vi "TextDiff.vi"(8 "error in (no error)":errorcluster, 9 "Output Folders":T5, 10 "VI 2 Screenshots in":T1, 11 "VI 1 Screenshots in":T1) -> (0 "error out":errorcluster, 2 "Description":string, 3 "appended path":path)   [LabVIEW 2020, in "VIDiffScreenshots.lvlib"]
uses:
  VIDiffScreenshots.lvlib
  Utilities/Output Folders.ctl
  VIScreenshots.ctl
  ScreenshotInfo.ctl
  Screenshot Type.ctl
  Utilities/FilePaths.ctl
  Utilities/VIDiffUtilities.lvlib
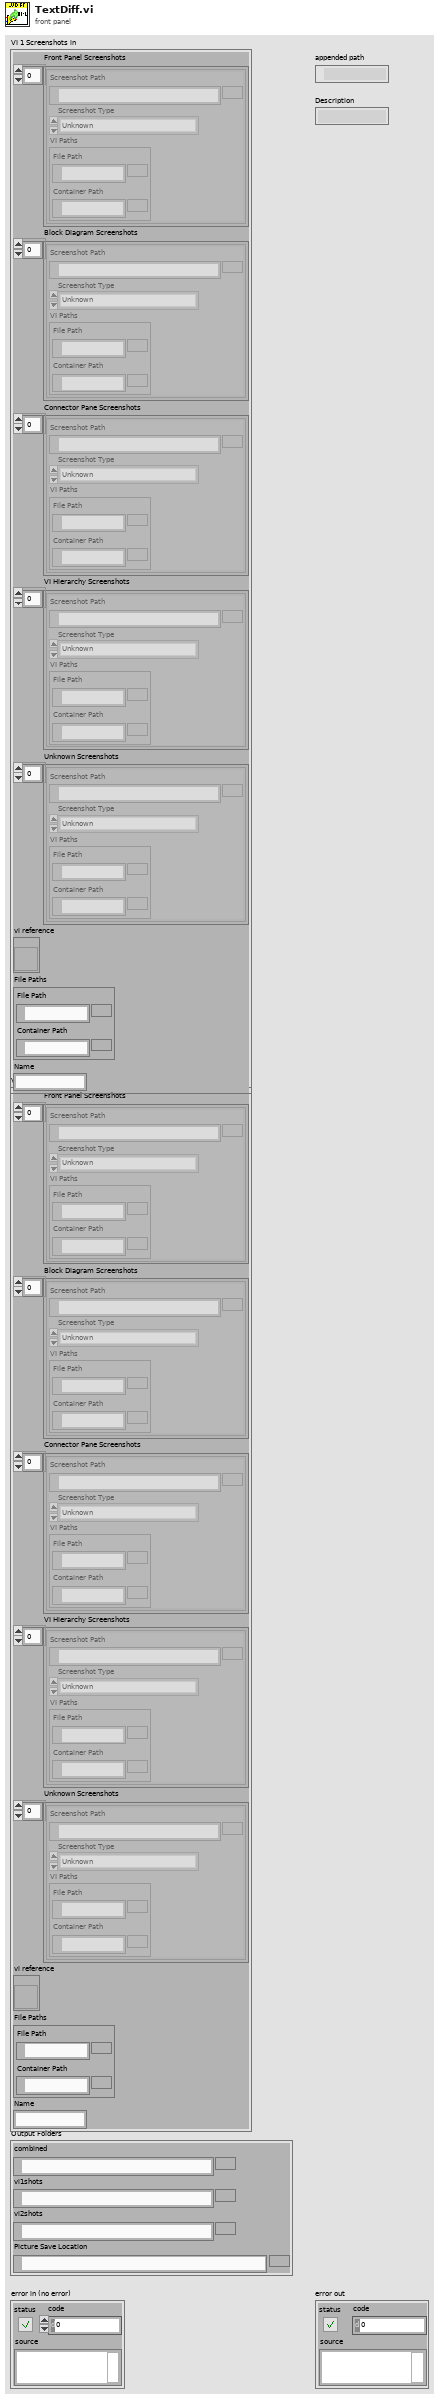
[diagram p1: front panel]
types:
  T1 = typedef "VIDiffScreenshots.lvlib/VIScreenshots.ctl" = cluster{"Front Panel Screenshots":T2[], "Block Diagram Screenshots":T2[], "Connector Pane Screenshots":T2[], "VI Hierarchy Screenshots":T2[], "Unknown Screenshots":T2[], "vi reference":refnum<vi>, "File Paths":cluster{"File Path":path, "Container Path":path}, "Name":string}
  T2 = typedef "VIDiffScreenshots.lvlib/ScreenshotInfo.ctl" = cluster{"Screenshot Path":path, "Screenshot Type":T3, "VI Paths":T4}
  T3 = typedef "VIDiffScreenshots.lvlib/Screenshot Type.ctl" = enum16{"Unknown", "Front Panel", "Connector Pane", "Block Diagram", "VI Hierarchy"}
  T4 = typedef "VIDiffUtilities.lvlib/FilePaths.ctl" = cluster{"File Path":path, "Container Path":path}
  T5 = typedef "VIDiffUtilities.lvlib/Output Folders.ctl" = cluster{"combined":path, "vi1shots":path, "vi2shots":path, "Picture Save Location":path}
  T6 = enum32{"invalid lock state", "Not Locked", "Locked (No Password)", "Password-protected"}
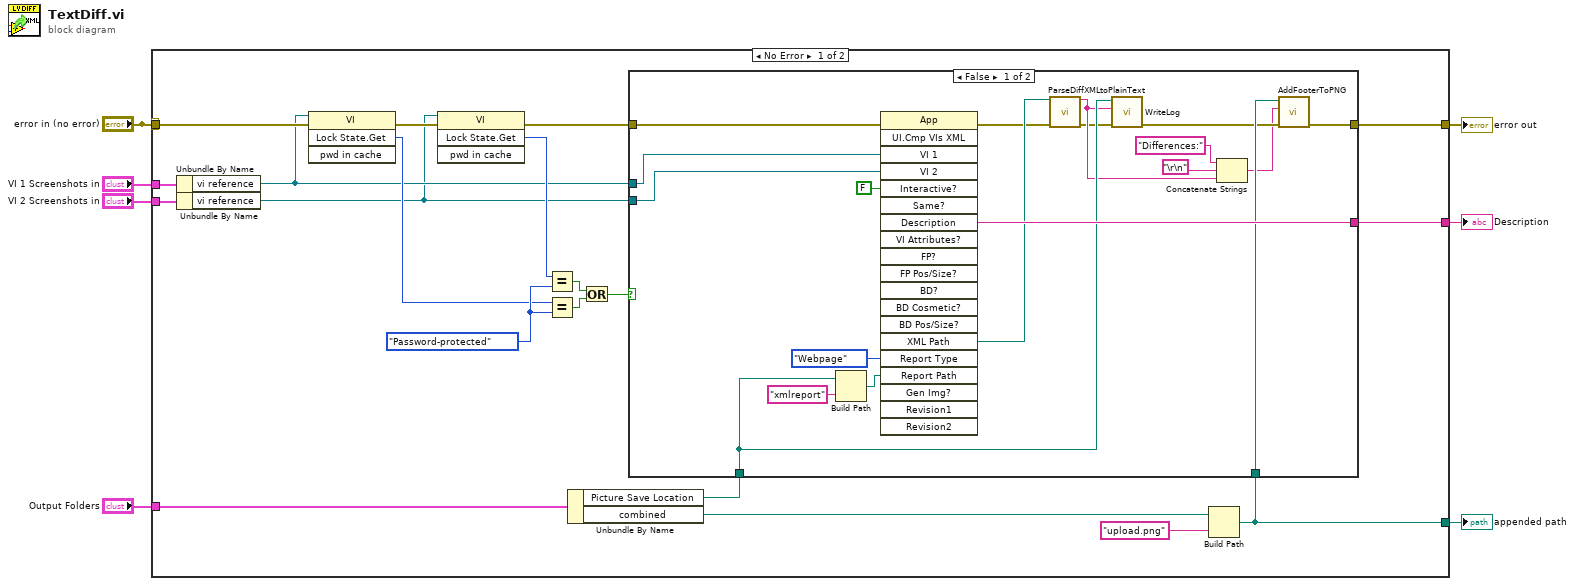
[diagram p0: block diagram]
diagram:
  n1 = case shown="No Error" "error in (no error)" {
    selector: "error in (no error)" -> [w21 w48]
    tunnel: "Output Folders" -> [w27 _]
    tunnel: "VI 2 Screenshots in" -> [w26 _]
    tunnel: "VI 1 Screenshots in" -> [w25 _]
    tunnel: "error in (no error)" -> [_ _]
    tunnel: [w24 _] -> w4
    tunnel: [w23 _] -> w3
    tunnel: [w22 w48] -> w2
    frame No Error {
      w18 = T6."Password-protected" ("y")
      n2 = Unbundle By Name(w25) -> ("vi reference"=w9:refnum<vi>)
      n3 = Unbundle By Name(w26) -> ("vi reference"=w8:refnum<vi>)
      n4 = invoke class="VI" method="Lock State.Get"(reference=w9, error in=w21) -> (error out=w19:errorcluster, "Get Lock State"=w14:T6)  [unwired: 2 in, 2 out]
      n5 = invoke class="VI" method="Lock State.Get"(reference=w8, error in=w19) -> (error out=w20:errorcluster, "Get Lock State"=w15:T6)  [unwired: 2 in, 2 out]
      n6 = Equal?(x=w15, y=w18) -> (x = y?=w16:bool)
      n7 = Equal?(x=w14, y=w18) -> (x = y?=w17:bool)
      n8 = Unbundle By Name(w27) -> ("Picture Save Location"=w12:path, "combined"=w13:path)
      n9 = Or(x=w16, y=w17) -> (x .or. y?=w10:bool)
      n10 = Build Path(base path=w13, name or relative path="upload.png") -> (appended path=w23:path)
      n11 = case shown="False" w10 {
        tunnel: [w46 _] -> w24
        tunnel: w23 -> [w45 _]
        tunnel: [w44 w47] -> w22
        tunnel: w20 -> [w43 w47]
        tunnel: w12 -> [w42 _]
        tunnel: w9 -> [w29 _]
        tunnel: w8 -> [w28 _]
        frame False {
          n12 = Build Path(base path=w42, name or relative path="xmlreport") -> (appended path=w40:path)
          n13 = invoke class="App" method="UI.Cmp VIs XML"(error in=w43, "VI 1"=w29, "VI 2"=w28, "Interactive?"=FALSE, "Report Type"=enum32{"None", "Webpage", "Text", "MS Word"}."Webpage", "Report Path"=w40) -> (error out=w33:errorcluster, "Description"=w46:string, "XML Path"=w41:path)  [unwired: 14 in, 17 out]
          n14 = call "ParseDiffXMLtoPlainText.vi"("XML Path"=w41, "error in"=w33) -> ("change description"=w36:string, "error out"=w34:errorcluster)  [unwired: 12 in]
          n15 = call "WriteLog.vi"("error in (no error)"=w34, "Log"=w36, "Log Folder"=w42) -> ("error out"=w35:errorcluster)  [unwired: 8 in]
          n16 = Concatenate Strings("Differences:" ("string"), "\r\n", w36) -> (w31:string)
          n17 = call "AddFooterToPNG.vi"("error in (no error)"=w35, "Footer String"=w31, "PNG File"=w45) -> ("error out"=w44:errorcluster)  [unwired: 8 in]
        }
        frame True {
          # "Can't get the XML for locked VIs"
        }
      }
    }
    frame Error {
    }
  }
  "Description" <- w4
  "appended path" <- w3
  "error out" <- w2
